vi "APC_9049_TS100ms_loop.vi"() -> ()   [LabVIEW 2020]
doc: "This example demonstrates the procedure required to apply different NI-DAQmx Custom Scales to each virtual channel in a task. A DAQmx Task Property Node (Functions >> NI Measurements >> DAQmx - Data Acquisition >> DAQmx Advanced Task Options) is used to obtain the task's virtual channels. A DAQmx Channel Property Node (Functions >> NI Measurements >> DAQmx - Data Acquisition) is then used to set the custom scale for each virtual channel in the task.\n\nThe \"DAQmx Create Scale\" VI creates a custom scale for each channel in the channel list. *Note, make sure your Minimum and Maximum channel parameters are consistent with the range the scale will create."
uses:
  <vilib>/Platform/TimedLoop/XDataNode/timing_clust.ctl
  <vilib>/Platform/TimedLoop/XDataNode/nitl_modes.ctl
  <vilib>/Platform/TimedLoop/XDataNode/wakeup.ctl
  <vilib>/addons/control/pid/pid.llb/PID Advanced (DBL Array).vi
  <vilib>/addons/control/pid/pid.llb/PID Parameter Manager (DBL Array).vi
  <vilib>/addons/control/pid/pid.llb/PID Derivative Action Buffered (DBL Array).vi
  <vilib>/addons/control/pid/pid.llb/PID Get Advanced Error (DBL Array).vi
  <vilib>/addons/control/pid/pid.llb/PID Integral Action Buffered (DBL Array).vi
  <vilib>/addons/control/pid/pid.llb/PID Resize 1D Array.vi
  <vilib>/addons/control/pid/pid.llb/PID Get Advanced Error (DBL).vi
  <vilib>/platform/TimedLoop/XDataNode/XDataNode.xnode
  <vilib>/Platform/TimedLoop/XDataNode/XDNodeRunTimeDep.lvlib
  <vilib>/addons/control/pid/NI_PID_pid.lvlib
panel:
  in  "learn control action?":bool[](array[boolean])=[FALSE, FALSE, FALSE, FALSE, FALSE, FALSE]
  out "dt out (s)":dbl format="%.3f"
  out "output":dbl[](array[numeric]) format="%.2f"
  in  "linearity":dbl[](array[numeric])=[1.0] format="%.2f"
  in  "beta":dbl[](array[numeric])=[1.0] format="%.2f"
  in  "reinitialize? (F)":bool
  in  "dt (s)":dbl=-1.0 format="%.3f"
  in  "PID gains":T1(array[cluster])=[{"proportional gain (Kc)"=1.0, "integral time (Ti, min)"=0.01, "derivative time (Td, min)"=0.0}, {"proportional gain (Kc)"=1.0, "integral time (Ti, min)"=0.01, "derivative time (Td, min)"=0.0}, {"proportional gain (Kc)"=1.0, "integral time (Ti, min)"=0.01, "derivative time (Td, min)"=0.0}, {"proportional gain (Kc)"=1.0, "integral time (Ti, min)"=0.01, "derivative time (Td, min)"=0.0}, {"proportional gain (Kc)"=1.0, "integral time (Ti, min)"=0.01, "derivative time (Td, min)"=0.0}, {"proportional gain (Kc)"=1.0, "integral time (Ti, min)"=0.01, "derivative time (Td, min)"=0.0}] {"derivative time (Td, min)" format="%.3f"; "integral time (Ti, min)" format="%.3f"; "proportional gain (Kc)" format="%.3f"}
  in  "setpoint range":T2(array[cluster])=[{"setpoint high"=100.0, "setpoint low"=0.0}, {"setpoint high"=100.0, "setpoint low"=0.0}, {"setpoint high"=100.0, "setpoint low"=0.0}, {"setpoint high"=100.0, "setpoint low"=0.0}, {"setpoint high"=100.0, "setpoint low"=0.0}, {"setpoint high"=100.0, "setpoint low"=0.0}] {"setpoint high" format="%.2f"; "setpoint low" format="%.2f"}
  in  "gamma":dbl[](array[numeric])=[0.0] format="%.2f"
  in  "process variable":dbl[](array[numeric])=[0.0] format="%.2f"
  in  "manual control":dbl[](array[numeric])=[0.0, 0.0, 0.0, 0.0, 0.0, 0.0] format="%.2f"
  in  "auto? (T)":bool[](array[boolean])=[FALSE, FALSE, FALSE, FALSE, FALSE, FALSE]
  in  "PID output range":cluster{"output high":dbl, "output low":dbl}[](array[cluster])=[{"output high"=100.0, "output low"=-100.0}, {"output high"=100.0, "output low"=-100.0}, {"output high"=100.0, "output low"=-100.0}, {"output high"=100.0, "output low"=-100.0}, {"output high"=100.0, "output low"=-100.0}, {"output high"=100.0, "output low"=-100.0}] {"output low" format="%.2f"; "output high" format="%.2f"}
  in  "setpoint":dbl[](array[numeric])=[0.0, 0.0, 0.0, 0.0, 0.0, 0.0] format="%.2f"
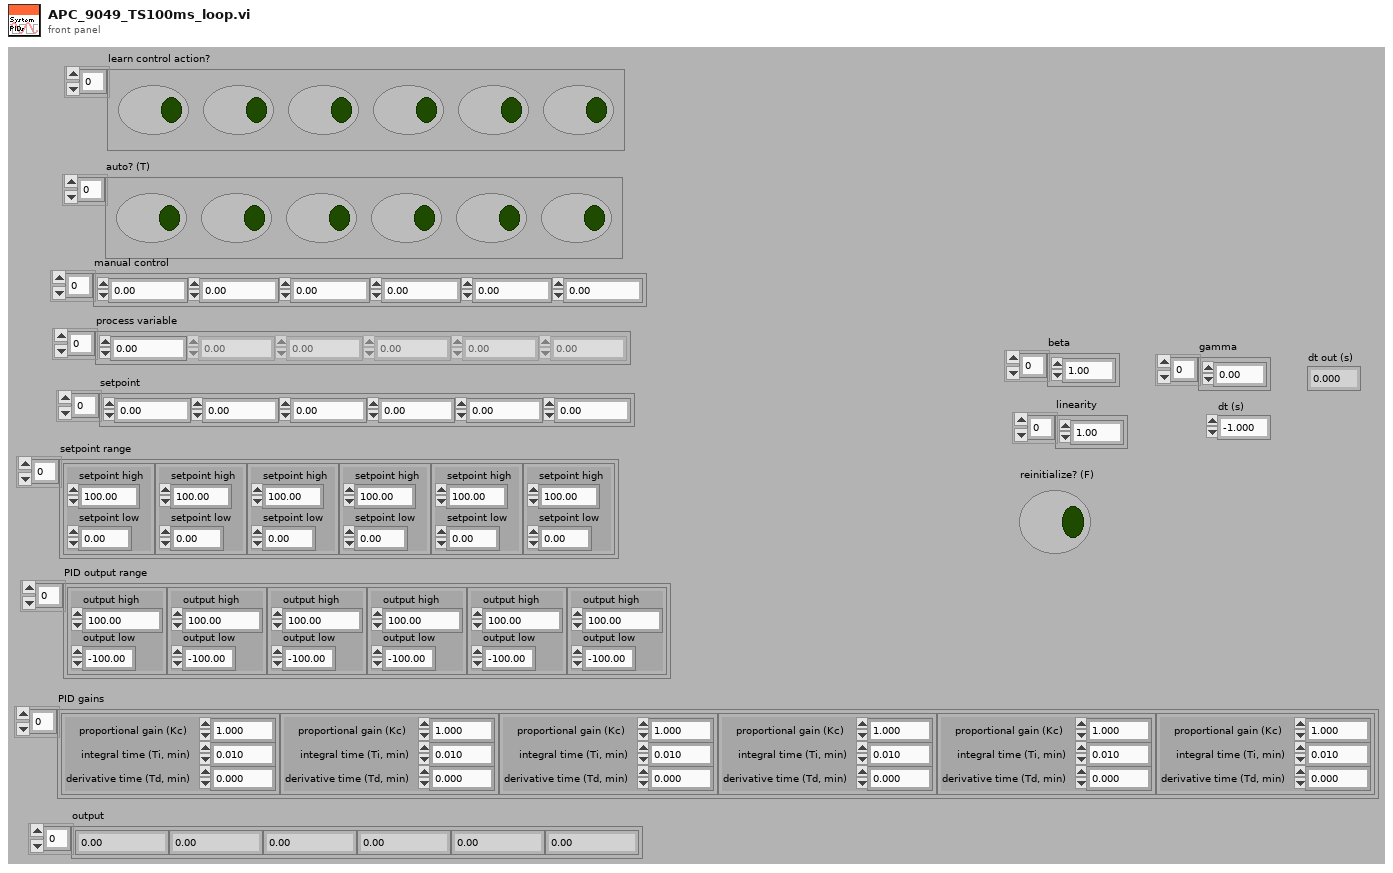
[diagram p1: front panel]
types:
  T1 = cluster{"proportional gain (Kc)":dbl, "integral time (Ti, min)":dbl, "derivative time (Td, min)":dbl}[]
  T2 = cluster{"setpoint high":dbl, "setpoint low":dbl}[]
  T3 = typedef "XDNodeRunTimeDep.lvlib/timing_clust.ctl" = cluster{"Expected End [f-1]":u64, "Actual End [f-1]":u64, "Finished Late? [f-1]":bool, "Expected End [i-1]":u64, "Actual End [i-1]":u64, "Finished Late? [i-1]":bool, "Expected Start [i]":u64, "Actual Start [i]":u64, "Expected Start [f]":u64, "Actual Start [f]":u64, "Source Name":string, "Structure Name":string, "Period":i64, "Deadline":i64, "Offset":i64, "Start":i64, "Priority":i32, "Timeout":i32, "Mode":T4, "Wakeup Reason":T5, "Error":errorcluster, "Source Type":string, "Secondary Source Type":string, "Global End Time":u64, "Global Start Time":u64, "Frame Duration":u64, "Iteration Duration":u64, "Assigned CPU":i32, "I/O Scan Engine Mode":u32}
  T4 = typedef "XDNodeRunTimeDep.lvlib/nitl_modes.ctl" = enum32{"No Change", "Process missed periods, maintain original phase", "Discard missed periods, maintain original phase", "Process missed periods, ignore original phase", "Discard missed periods, ignore original phase"}
  T5 = typedef "XDNodeRunTimeDep.lvlib/wakeup.ctl" = enum32{"Normal", "Aborted", "Asynchronous wakeup", "Timing source error", "Timed loop error", "Timeout"}
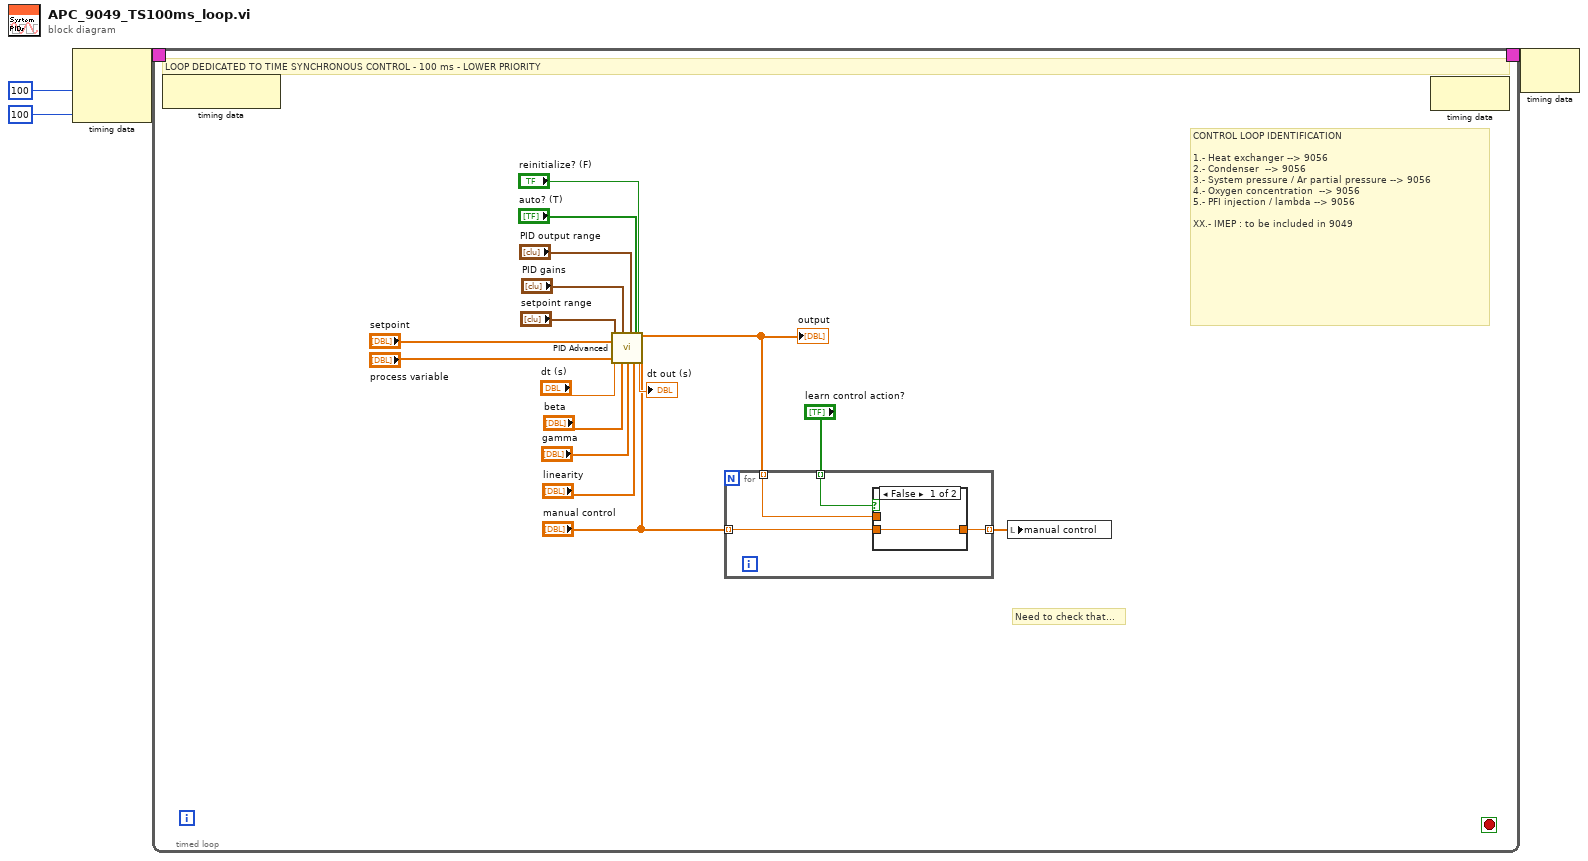
[diagram p0: block diagram]
diagram:
  n1 = node-c288(i64 100 ("Period"), 100 ("Priority")) -> (w4:T3)  [unwired: 1 in]
  n2 = timed-loop {
    timing: w4 -> [_]
    timing-out: [_] -> w3
    stop <- _ stop-if-true
    # "CONTROL LOOP IDENTIFICATION\n\n1.- Heat exchanger --> 9056\n2.- Condenser  --> 9056\n3.- System pressure / Ar partial pressure --> 9056\n4.- Oxygen concentration  --> 9056\n5.- PFI injection / lambda --> 9056\n\nXX.- IMEP : to be included in 9049"
    # "Need to check that..."
    # "LOOP DEDICATED TO TIME SYNCHRONOUS CONTROL - 100 ms - LOWER PRIORITY"
    n3 = node-c288() -> ()  [unwired: 1 in, 1 out]
    n4 = call-poly <vilib>:"PID Advanced.vi"("setpoint"="setpoint", "output range"="PID output range", "auto? (T)"="auto? (T)", "manual control"="manual control", "process variable"="process variable", "gamma"="gamma", "setpoint range"="setpoint range", "PID gains"="PID gains", "dt (s)"="dt (s)", "reinitialize? (F)"="reinitialize? (F)", "beta"="beta", "linearity"="linearity") -> ("output"=w7:dbl[], "dt out (s)"=→"dt out (s)":dbl)  [unwired: 2 in]
    "output" <- w7
    n5 = for {
      tunnel: "learn control action?" -> [w24] mode=indexing
      tunnel: w7 -> [w23] mode=indexing
      tunnel: "manual control" -> [w22] mode=indexing
      tunnel: [w21] -> w5 mode=indexing
      n6 = case shown="False" w24 {
        tunnel: w23 -> [_ w26]
        tunnel: w22 -> [w25 _]
        tunnel: [w25 w26] -> w21
        frame False {
        }
        frame True {
        }
      }
    }
    n7 = local write "manual control"(w5) -> ()
    n8 = node-c288() -> ()  [unwired: 1 in, 1 out]
  }
  n9 = node-c288(w3) -> ()  [unwired: 1 out]
